vi "Debug.vi"   [LabVIEW 2012]
uses:
  <vilib>/Rock Robotics/WPI/Solenoid/WPI_SolenoidValue.ctl
  <vilib>/Rock Robotics/WPI/Relay/WPI_RelayValue.ctl
  Robot Global Data.vi
  <vilib>/Rock Robotics/WPI/Joystick/WPI_JoystickGetSetRefNum.vi
  <vilib>/Rock Robotics/WPI/Solenoid/WPI_SolenoidSetEnum.vi
  <vilib>/Rock Robotics/WPI/RobotDrive/WPI_RobotDriveGetSetRefNum.vi
types:
  T1 = typedef "WPI_JoystickDevRef.ctl" = cluster{"Device":T2}
  T2 = typedef "WPI_JoystickDeviceEnum.ctl" = enum16{"USB 1", "USB 2", "USB 3", "USB 4", "Kinect 1", "Kinect 2"}
  T3 = typedef "WPI_JoystickButtonState.ctl" = cluster{"Button 1":bool, "Button 2":bool, "Button 3":bool, "Button 4":bool, "Button 5":bool, "Button 6":bool, "Button 7":bool, "Button 8":bool, "Button 9":bool, "Button 10":bool, "Button 11":bool, "Button 12":bool}
  T4 = cluster{"axis 1 (x)":dbl, "axis 2 (y)":dbl, "axis 3 (throttle)":dbl, "axis 4":dbl, "axis 5":dbl, "axis 6":dbl}
  T5 = typedef "WPI_RobotDriveDevRef.ctl" = cluster{"DevStatus":errorcluster, "Motors[]":T6[], "Square Inputs":bool, "Max Output":dbl, "Isochronous":bool}
  T6 = typedef "WPI_MotorControlDeviceRef.ctl" = cluster{"DeviceStatus":errorcluster, "Type":enum16{"PWM", "CAN"}, "PWM":cluster{"Digital Module":T7, "PWM Channel":T8, "DeadBand":T9}, "CAN":cluster{"Device Number":u8, "Control Mode":T10, "Semaphore":T11, "Max Vout":dbl}, "Invert":bool, "TransformRef":T12, "InvTransformRef":T12}
  T7 = typedef "FPGA_TypedefDigitalModule.ctl" = enum16{"Digital Module 1", "Digital Module 2"}
  T8 = typedef "FPGA_DIOPWMChannel.ctl" = enum8{"PWM 1", "PWM 2", "PWM 3", "PWM 4", "PWM 5", "PWM 6", "PWM 7", "PWM 8", "PWM 9", "PWM 10", "Invalid"}
  T9 = typedef "WPI_PWMDeadband.ctl" = cluster{"Name":string, "maxPositivePwm":i32, "minPositivePwm":i32, "centerPwm":i32, "maxNegativePwm":i32, "minNegativePwm":i32, "angularRange":u16}
  T10 = typedef "WPI_CANJaguar_ControlMode.ctl" = enum8{"Percent VBus", "Current", "Speed", "Position", "Voltage"}
  T11 = typedef "Semaphore RefNum" = refnum<k1>
  T12 = typedef "WPI_PWMTransform_ConPane.ctl" = refnum<vi>
  T13 = typedef "WPI_RelayValue.ctl" = enum16{"Off", "On", "Forward", "Reverse"}
  T14 = typedef "WPI_RelayDevRef.ctl" = cluster{"DevStatus":errorcluster, "Relay Channel":T15, "Digital Module":T7, "Relay Direction":T16}
  T15 = typedef "FPGA_DIORelayChannel.ctl" = enum8{"Relay 1", "Relay 2", "Relay 3", "Relay 4", "Relay 5", "Relay 6", "Relay 7", "Relay 8", "Invalid"}
  T16 = typedef "WPI_RelayDirection.ctl" = enum16{"Both directions", "Forward only", "Reverse only"}
  T17 = typedef "WPI_SolenoidValue.ctl" = enum16{"Off", "On", "Forward", "Reverse"}
  T18 = typedef "WPI_SolenoidDevRef.ctl" = cluster{"DevStatus":errorcluster, "Solenoid Module":T19, "Forward Solenoid Channel":T20, "Reverse Solenoid Channel":T20}
  T19 = typedef "FPGA_TypedefSolenoidModule.ctl" = enum16{"Solenoid Module 1", "Solenoid Module 2"}
  T20 = typedef "WPI_SolenoidChannel.ctl" = enum8{"Solenoid 1", "Solenoid 2", "Solenoid 3", "Solenoid 4", "Solenoid 5", "Solenoid 6", "Solenoid 7", "Solenoid 8", "Invalid"}
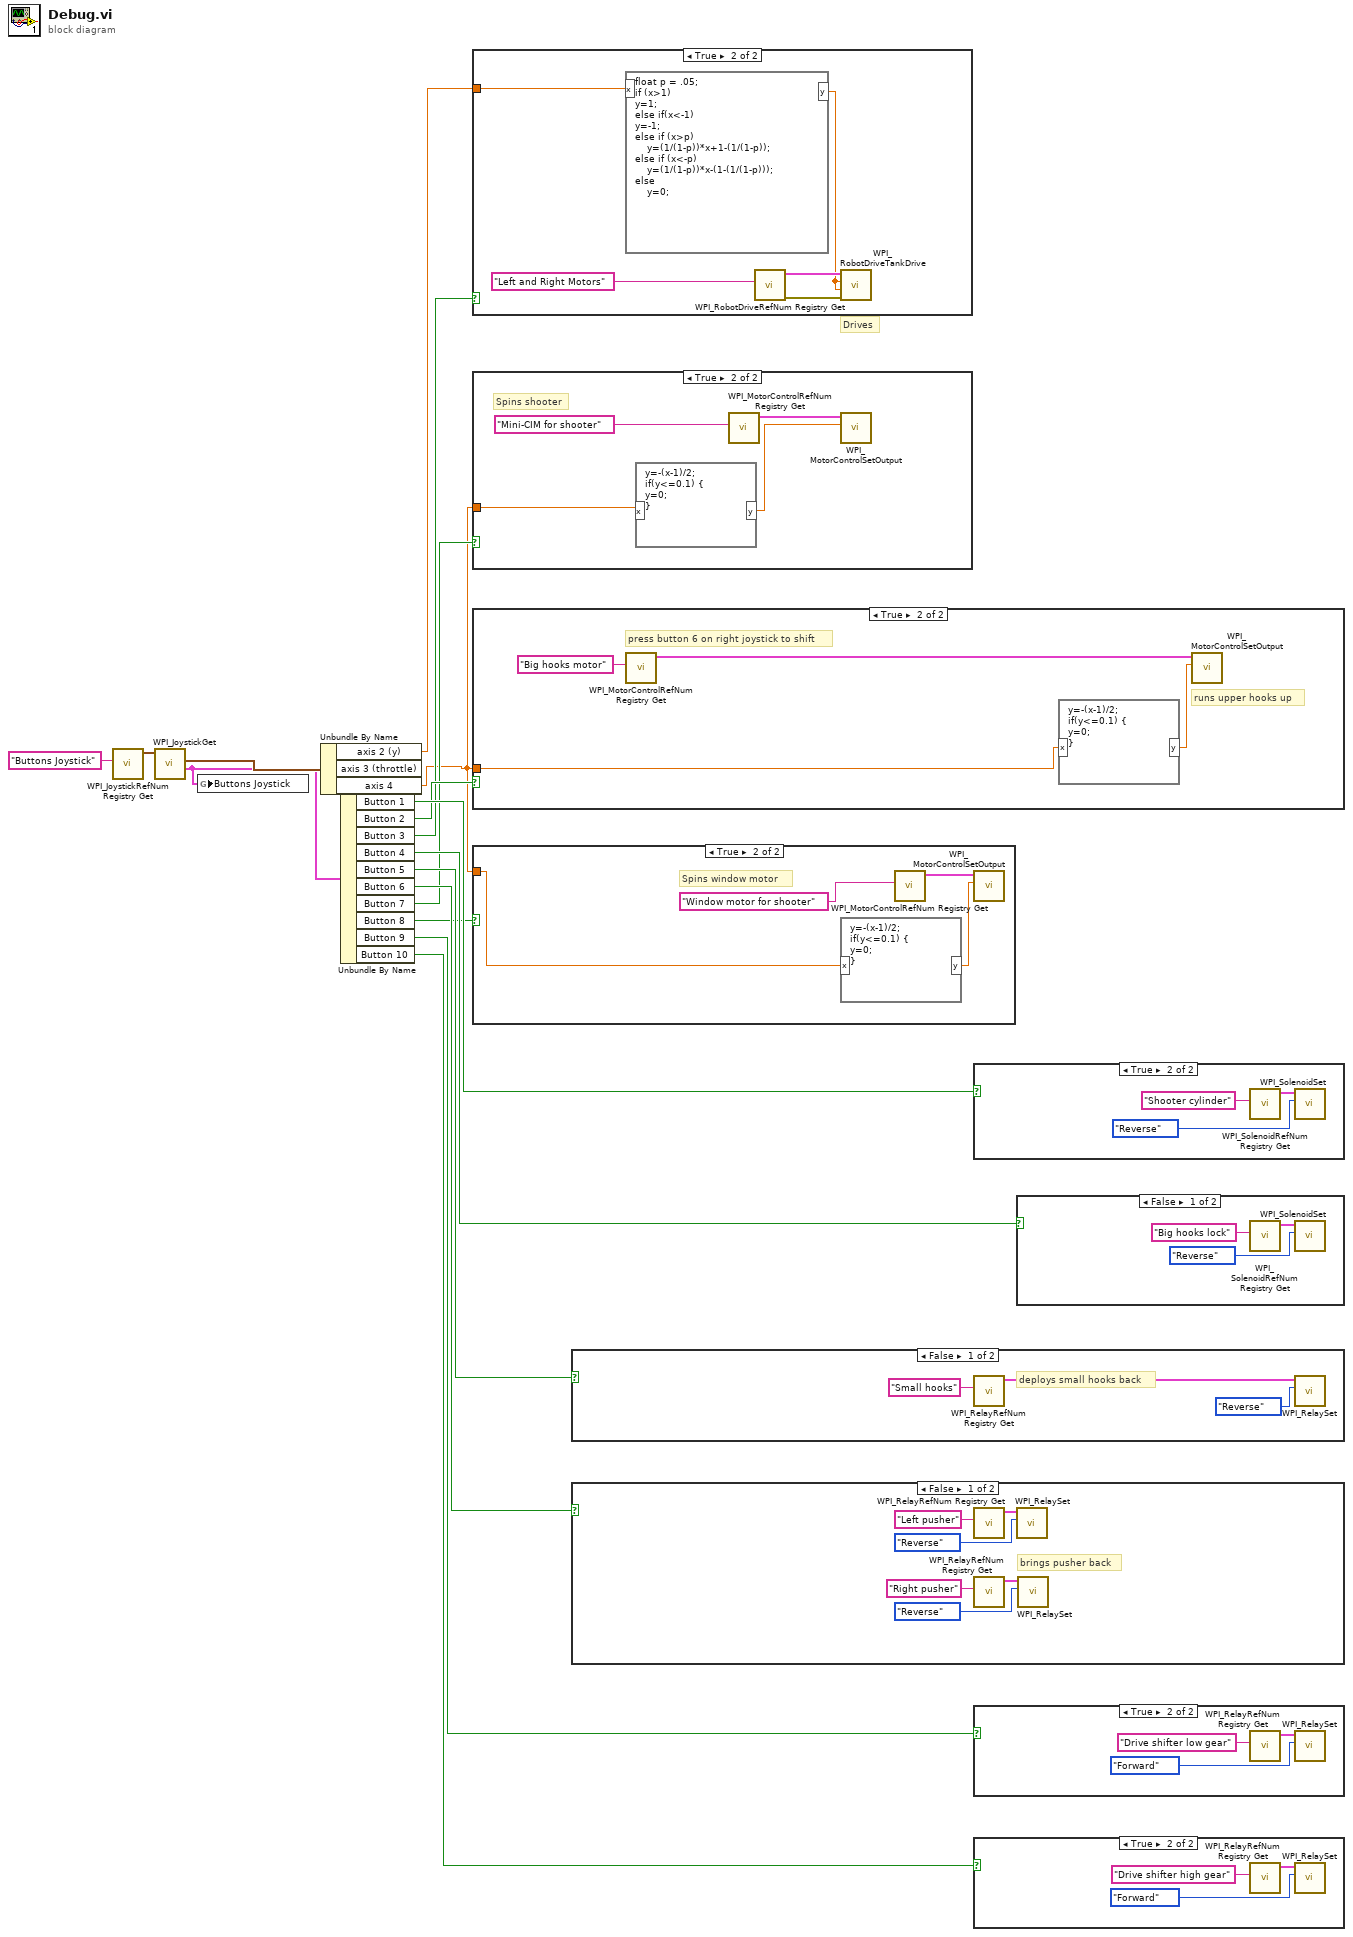
[diagram p0: block diagram]
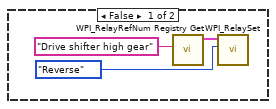
[diagram p2: hidden frame]
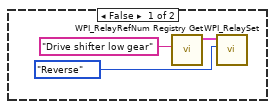
[diagram p3: hidden frame]
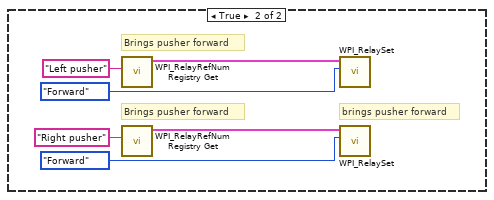
[diagram p6: hidden frame]
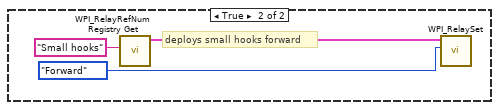
[diagram p7: hidden frame]
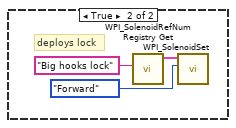
[diagram p8: hidden frame]
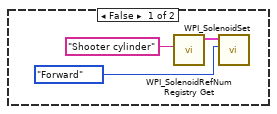
[diagram p11: hidden frame]
diagram:
  # "Drives"
  n1 = call <vilib>:"WPI_JoystickRefNum Registry Get.vi"("refnum name"="Buttons Joystick") -> ("JoystickDevRef"=w16:T1)  [unwired: 1 in, 9 out]
  n2 = call <vilib>:"WPI_JoystickGet.vi"("JoystickDevRef"=w16) -> ("Buttons"=w13:T3, "Axes"=w14:T4)  [unwired: 1 in, 4 out]
  n3 = global write "Robot Global Data.vi" "Buttons Joystick"(w13) -> ()
  n4 = Unbundle By Name(w14) -> ("axis 2 (y)"=w9:dbl, "axis 4"=w1:dbl)  [unwired: 1 out]
  n5 = Unbundle By Name(w13) -> ("Button 1"=w12:bool, "Button 2"=w11:bool, "Button 3"=w10:bool, "Button 4"=w8:bool, "Button 5"=w7:bool, "Button 6"=w6:bool, "Button 7"=w5:bool, "Button 8"=w4:bool, "Button 9"=w3:bool, "Button 10"=w2:bool)
  n6 = case shown="True" w10 {
    tunnel: w9 -> [_ w18]
    frame False {
    }
    frame True {
      n7 = formula code="float p = .05; \nif (x>1)\ny=1;\nelse if(x<-1)\ny=-1;\nelse if (x>p)\n    y=(1/(1-p))*x+1-(1/(1-p));\nelse if (x<-p) \n    y=(1/(1-p))*x-(1-(1/(1-p)));\nelse\n    y=0;"("x"=w18) -> ("y"=w17:dbl)
      n8 = call <vilib>:"WPI_RobotDriveRefNum Registry Get.vi"("refnum name"="Left and Right Motors") -> ("error out"=w21:errorcluster, "RobotDriveDevRef"=w20:T5)  [unwired: 1 in, 8 out]
      n9 = call <vilib>:"WPI_RobotDriveTankDrive.vi"("error in (no error)"=w21, "Right axis value"=w17, "Left axis value"=w17, "RobotDriveDevRef"=w20) -> ()  [unwired: 5 in, 3 out]
    }
  }
  n10 = case shown="True" w5 {
    tunnel: w1 -> [_ w23]
    frame False {
    }
    frame True {
      # "Spins shooter"
      n11 = formula code="y=-(x-1)/2;\nif(y<=0.1) {\ny=0;\n}"("x"=w23) -> ("y"=w22:dbl)
      n12 = call <vilib>:"WPI_MotorControlRefNum Registry Get.vi"("refnum name"="Mini-CIM for shooter") -> ("MotorControlDevRef"=w24:T6)  [unwired: 9 in, 1 out]
      n13 = call <vilib>:"WPI_MotorControlSetOutput.vi"("Output"=w22, "MotorControlDevRef"=w24) -> ()  [unwired: 7 in, 3 out]
    }
  }
  n14 = case shown="True" w11 {
    tunnel: w1 -> [_ w27]
    frame False {
    }
    frame True {
      # "press button 6 on right joystick to shift"
      # "runs upper hooks up"
      n15 = call <vilib>:"WPI_MotorControlRefNum Registry Get.vi"("refnum name"="Big hooks motor") -> ("MotorControlDevRef"=w28:T6)  [unwired: 9 in, 1 out]
      n16 = formula code="y=-(x-1)/2;\nif(y<=0.1) {\ny=0;\n}"("x"=w27) -> ("y"=w26:dbl)
      n17 = call <vilib>:"WPI_MotorControlSetOutput.vi"("Output"=w26, "MotorControlDevRef"=w28) -> ()  [unwired: 7 in, 3 out]
    }
  }
  n18 = case shown="True" w4 {
    tunnel: w1 -> [_ w31]
    frame False {
    }
    frame True {
      # "Spins window motor"
      n19 = formula code="y=-(x-1)/2;\nif(y<=0.1) {\ny=0;\n}"("x"=w31) -> ("y"=w30:dbl)
      n20 = call <vilib>:"WPI_MotorControlRefNum Registry Get.vi"("refnum name"="Window motor for shooter") -> ("MotorControlDevRef"=w32:T6)  [unwired: 9 in, 1 out]
      n21 = call <vilib>:"WPI_MotorControlSetOutput.vi"("Output"=w30, "MotorControlDevRef"=w32) -> ()  [unwired: 7 in, 3 out]
    }
  }
  n22 = case shown="False" w7 {
    frame False {
      # "deploys small hooks back"
      n23 = call <vilib>:"WPI_RelayRefNum Registry Get.vi"("refnum name"="Small hooks") -> ("RelayDevRef"=w36:T14)  [unwired: 9 in, 1 out]
      n24 = call <vilib>:"WPI_RelaySet.vi"("RelayValue"=WPI_RelayValue."Reverse", "RelayDevRef"=w36) -> ()  [unwired: 8 in, 2 out]
    }
    frame True {
      # "deploys small hooks forward"
      n25 = call <vilib>:"WPI_RelayRefNum Registry Get.vi"("refnum name"="Small hooks") -> ("RelayDevRef"=w39:T14)  [unwired: 9 in, 1 out]
      n26 = call <vilib>:"WPI_RelaySet.vi"("RelayValue"=WPI_RelayValue."Forward", "RelayDevRef"=w39) -> ()  [unwired: 8 in, 2 out]
    }
  }
  n27 = case shown="False" w6 {
    frame False {
      # "brings pusher back"
      n28 = call <vilib>:"WPI_RelayRefNum Registry Get.vi"("refnum name"="Left pusher") -> ("RelayDevRef"=w45:T14)  [unwired: 9 in, 1 out]
      n29 = call <vilib>:"WPI_RelayRefNum Registry Get.vi"("refnum name"="Right pusher") -> ("RelayDevRef"=w42:T14)  [unwired: 9 in, 1 out]
      n30 = call <vilib>:"WPI_RelaySet.vi"("RelayValue"=WPI_RelayValue."Reverse", "RelayDevRef"=w45) -> ()  [unwired: 8 in, 2 out]
      n31 = call <vilib>:"WPI_RelaySet.vi"("RelayValue"=WPI_RelayValue."Reverse", "RelayDevRef"=w42) -> ()  [unwired: 8 in, 2 out]
    }
    frame True {
      # "brings pusher forward"
      # "Brings pusher forward"
      # "Brings pusher forward"
      n32 = call <vilib>:"WPI_RelayRefNum Registry Get.vi"("refnum name"="Left pusher") -> ("RelayDevRef"=w51:T14)  [unwired: 9 in, 1 out]
      n33 = call <vilib>:"WPI_RelayRefNum Registry Get.vi"("refnum name"="Right pusher") -> ("RelayDevRef"=w48:T14)  [unwired: 9 in, 1 out]
      n34 = call <vilib>:"WPI_RelaySet.vi"("RelayValue"=WPI_RelayValue."Forward", "RelayDevRef"=w51) -> ()  [unwired: 8 in, 2 out]
      n35 = call <vilib>:"WPI_RelaySet.vi"("RelayValue"=WPI_RelayValue."Forward", "RelayDevRef"=w48) -> ()  [unwired: 8 in, 2 out]
    }
  }
  n36 = case shown="True" w12 {
    frame False {
      n37 = call <vilib>:"WPI_SolenoidRefNum Registry Get.vi"("refnum name"="Shooter cylinder") -> ("SolenoidDevRef"=w53:T18)  [unwired: 9 in, 1 out]
      n38 = call-poly <vilib>:"WPI_SolenoidSet.vi"("Value"=WPI_SolenoidValue."Forward", "SolenoidDevRef"=w53) -> ()  [unwired: 8 in, 2 out]
    }
    frame True {
      n39 = call <vilib>:"WPI_SolenoidRefNum Registry Get.vi"("refnum name"="Shooter cylinder") -> ("SolenoidDevRef"=w56:T18)  [unwired: 9 in, 1 out]
      n40 = call-poly <vilib>:"WPI_SolenoidSet.vi"("Value"=WPI_SolenoidValue."Reverse", "SolenoidDevRef"=w56) -> ()  [unwired: 8 in, 2 out]
    }
  }
  n41 = case shown="True" w3 {
    frame False {
      n42 = call <vilib>:"WPI_RelayRefNum Registry Get.vi"("refnum name"="Drive shifter low gear") -> ("RelayDevRef"=w60:T14)  [unwired: 9 in, 1 out]
      n43 = call <vilib>:"WPI_RelaySet.vi"("RelayValue"=WPI_SolenoidValue."Reverse" ("Value"), "RelayDevRef"=w60) -> ()  [unwired: 8 in, 2 out]
    }
    frame True {
      n44 = call <vilib>:"WPI_RelayRefNum Registry Get.vi"("refnum name"="Drive shifter low gear") -> ("RelayDevRef"=w63:T14)  [unwired: 9 in, 1 out]
      n45 = call <vilib>:"WPI_RelaySet.vi"("RelayValue"=WPI_SolenoidValue."Forward" ("Value"), "RelayDevRef"=w63) -> ()  [unwired: 8 in, 2 out]
    }
  }
  n46 = case shown="True" w2 {
    frame False {
      n47 = call <vilib>:"WPI_RelayRefNum Registry Get.vi"("refnum name"="Drive shifter high gear") -> ("RelayDevRef"=w66:T14)  [unwired: 9 in, 1 out]
      n48 = call <vilib>:"WPI_RelaySet.vi"("RelayValue"=WPI_SolenoidValue."Reverse" ("Value"), "RelayDevRef"=w66) -> ()  [unwired: 8 in, 2 out]
    }
    frame True {
      n49 = call <vilib>:"WPI_RelayRefNum Registry Get.vi"("refnum name"="Drive shifter high gear") -> ("RelayDevRef"=w69:T14)  [unwired: 9 in, 1 out]
      n50 = call <vilib>:"WPI_RelaySet.vi"("RelayValue"=WPI_SolenoidValue."Forward" ("Value"), "RelayDevRef"=w69) -> ()  [unwired: 8 in, 2 out]
    }
  }
  n51 = case shown="False" w8 {
    frame False {
      n52 = call <vilib>:"WPI_SolenoidRefNum Registry Get.vi"("refnum name"="Big hooks lock") -> ("SolenoidDevRef"=w71:T18)  [unwired: 9 in, 1 out]
      n53 = call-poly <vilib>:"WPI_SolenoidSet.vi"("Value"=WPI_SolenoidValue."Reverse", "SolenoidDevRef"=w71) -> ()  [unwired: 8 in, 2 out]
    }
    frame True {
      # "deploys lock"
      n54 = call <vilib>:"WPI_SolenoidRefNum Registry Get.vi"("refnum name"="Big hooks lock") -> ("SolenoidDevRef"=w74:T18)  [unwired: 9 in, 1 out]
      n55 = call-poly <vilib>:"WPI_SolenoidSet.vi"("Value"=WPI_SolenoidValue."Forward", "SolenoidDevRef"=w74) -> ()  [unwired: 8 in, 2 out]
    }
  }
